vi "Configure Filters.vi"(7 "Virtual Memory Unit in":refnum<class "Virtual Memory Unit.lvclass">, 8 "error in (no error)":errorcluster, 11 "Bus Monitor in":refnum<class "Bus Monitor.lvclass">) -> (0 "error out":errorcluster, 3 "Bus Monitor out":refnum<class "Bus Monitor.lvclass">, 5 "Virtual Memory Unit out":refnum<class "Virtual Memory Unit.lvclass">)   [LabVIEW 2020, in "BCI-1553 API.lvlib" / "Bus Monitor.lvclass"]
uses:
  Bus Monitor.lvclass
  Dependencies/Virtual Memory Unit/Virtual Memory Unit.lvclass
  Bus Monitor.lvclass/Bus Monitor.ctl
  Dependencies/Registry/Registry.lvclass/Registry.ctl
  Filters/Filter/Filter.lvclass
  Dependencies/Registry/Registry.lvclass
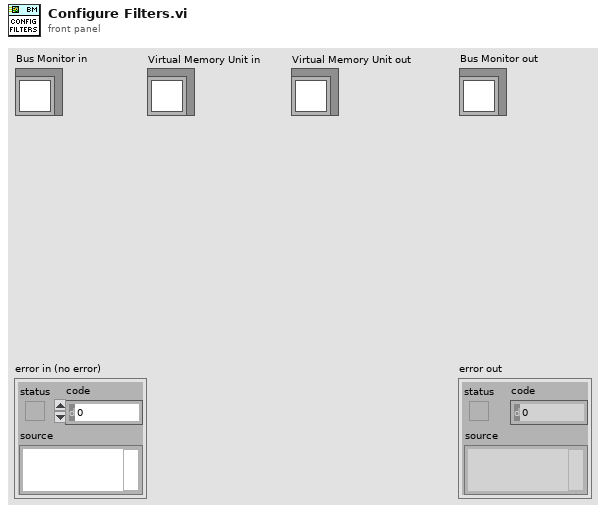
[diagram p1: front panel]
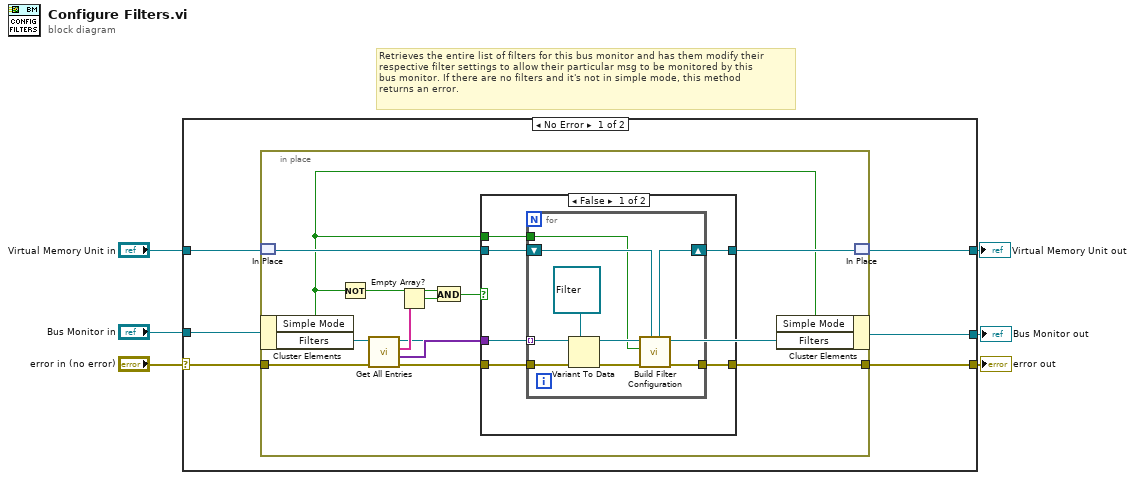
[diagram p0: block diagram]
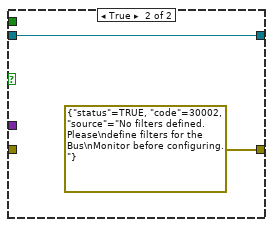
[diagram p2: hidden frame]
diagram:
  # "Retrieves the entire list of filters for this bus monitor and has them modify their\nrespective filter settings to allow their particular msg to be monitored by this\nbus monitor. If there are no filters and it's not in simple mode, this method\nreturns an error."
  n1 = case shown="No Error" "error in (no error)" {
    selector: "error in (no error)" -> [w10 w44]
    tunnel: [w9 w44] -> w5
    tunnel: [w11 w43] -> w3
    tunnel: "Bus Monitor in" -> [w12 w43]
    tunnel: [w7 w42] -> w2
    tunnel: "Virtual Memory Unit in" -> [w8 w42]
    frame No Error {
      n2 = in-place {
        in-place-border: w10 -> [w24]
        in-place-border: [w17] -> w9
        n3 = in-place-match #1(w8) -> (w21:refnum<class "Virtual Memory Unit.lvclass">)
        n4 = in-place-cluster #2(w12) -> ("Simple Mode"=w13:bool, "Filters"=w18:refnum<class "Registry.lvclass">)
        n5 = Not(x=w13) -> (.not. x?=w14:bool)
        n6 = call "Get All Entries.vi"("error in (no error)"=w24, "Registry in"=w18) -> ("error out"=w23:errorcluster, "Values"=w22:variant[], "Keys"=w20:string[])  [unwired: 7 in]
        n7 = Empty Array?(array=w20) -> (empty?=w16:bool)
        n8 = And(x=w14, y=w16) -> (x .and. y?=w15:bool)
        n9 = case shown="False" w15 {
          tunnel: w23 -> [w30 _]
          tunnel: w22 -> [w29 _]
          tunnel: w21 -> [w28 w41]
          tunnel: [w27 w41] -> w19
          tunnel: [w26 errorcluster {"status"=TRUE, "code"=30002, "source"="No filters defined. Please\ndefine filters for the Bus\nMonitor before configuring."} ("error out")] -> w17
          tunnel: w13 -> [w25 _]
          frame False {
            n10 = for {
              tunnel: w30 -> [w39]
              tunnel: w29 -> [w38] mode=indexing
              shift-right: [w33] -> w27
              shift-left: w28 -> [w34]
              tunnel: [w32] -> w26
              tunnel: w25 -> [w31]
              n11 = Variant To Data(error in=w39, type=refnum<class "Filter.lvclass"> refnum ("SLSC 1553 API.lvlib:Filter.lvclass"), Variant=w38) -> (data=w36:refnum<class "Filter.lvclass">, error out=w35:errorcluster)
              n12 = call-dynamic "Build Filter Configuration.vi"("Virtual Memory Unit in"=w34, "error in (no error)"=w35, "Simple Mode (Blacklist)"=w31, "Filter in"=w36) -> ("error out"=w32:errorcluster, "Virtual Memory Unit out"=w33:refnum<class "Virtual Memory Unit.lvclass">)  [unwired: 6 in]
            }
          }
          frame True {
          }
        }
        n13 = in-place-cluster #2("Simple Mode"=w13, "Filters"=w18) -> (w11:refnum<class "Bus Monitor.lvclass">)
        n14 = in-place-match #1(w19) -> (w7:refnum<class "Virtual Memory Unit.lvclass">)
      }
    }
    frame Error {
    }
  }
  "error out" <- w5
  "Bus Monitor out" <- w3
  "Virtual Memory Unit out" <- w2
